vi "Set Bucket Versioning.vi"(6 "Auth device data":T1, 7 "Versioning Configuration":T2={"Status"=enum."Suspended", "MfaDelete"=enum."Disabled"}, 8 "error in (no error)":errorcluster, 9 "Bucket":string) -> (0 "error out":errorcluster)   [LabVIEW 2011, in "LV Interface for Amazon S3.lvlib"]
doc: "This operation <B>sets the versioning state of an existing bucket</B>. To set the versioning state, you <B>must be the bucket owner</B>."
uses:
  LV Interface for Amazon S3.lvlib
  Typedefs/AMZ_S3_API_VersioningConfiguration.ctl
  Typedefs/AMZ_S3_Versioning Status.ctl
  Typedefs/AMZ_S3_MFA Delete.ctl
  Typedefs/AMZ_S3_Auth Device Data.ctl
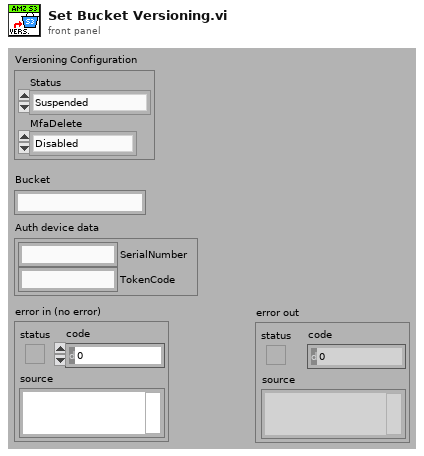
[diagram p1: front panel]
types:
  T1 = typedef "LV Interface for Amazon S3.lvlib/AMZ_S3_Auth Device Data.ctl" = cluster{"SerialNumber":string, "TokenCode":string}
  T2 = typedef "LV Interface for Amazon S3.lvlib/AMZ_S3_API_VersioningConfiguration.ctl" = cluster{"Status":T3, "MfaDelete":T4}
  T3 = typedef "LV Interface for Amazon S3.lvlib/AMZ_S3_Versioning Status.ctl" = enum16{"Disabled", "Suspended", "Enabled"}
  T4 = typedef "LV Interface for Amazon S3.lvlib/AMZ_S3_MFA Delete.ctl" = enum16{"Disabled", "Enabled"}
  T5 = typedef "LV Interface for Amazon S3.lvlib/AMZ_S3_HTTP Header-Value pair.ctl" = cluster{"Header":string, "Value":string}
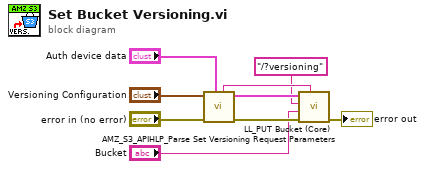
[diagram p0: block diagram]
diagram:
  n1 = call "AMZ_S3_APIHLP_Parse Set Versioning Request Parameters.vi"("Auth device data"="Auth device data", "error in (no error)"="error in (no error)", "VersioningConfiguration"="Versioning Configuration") -> ("error out"=w6:errorcluster, "HTTP Headers"=w5:T5[], "PUT Data"=w4:string)  [unwired: 6 in]
  n2 = call "LL_PUT Bucket (Core).vi"("Data"=w4, "error in (no error)"=w6, "Bucket"="Bucket", "Path and query string"="/?versioning", "Headers"=w5) -> ("error out"=→"error out":errorcluster)  [unwired: 3 in, 3 out]
